vi "Untitled 1.vi"() -> ()   [LabVIEW 2024]
uses:
  <vilib>/DAQmx/read.llb/DAQmx Read (Analog 1D Wfm NChan NSamp).vi
  <vilib>/addons/database/Connection.llb/DB Tools Open Connec (Path).vi
  <vilib>/Utility/file.llb/Write Delimited Spreadsheet (DBL).vi
  <vilib>/DAQmx/miscellaneous.llb/DAQmx Fill In Error Info.vi
  <vilib>/addons/database/NI_Database_API.lvlib
panel:
  out "overflow element":dbl[][](array[numeric])
  out "error out":errorcluster
  in  "connection information":path
  in  "stop":bool
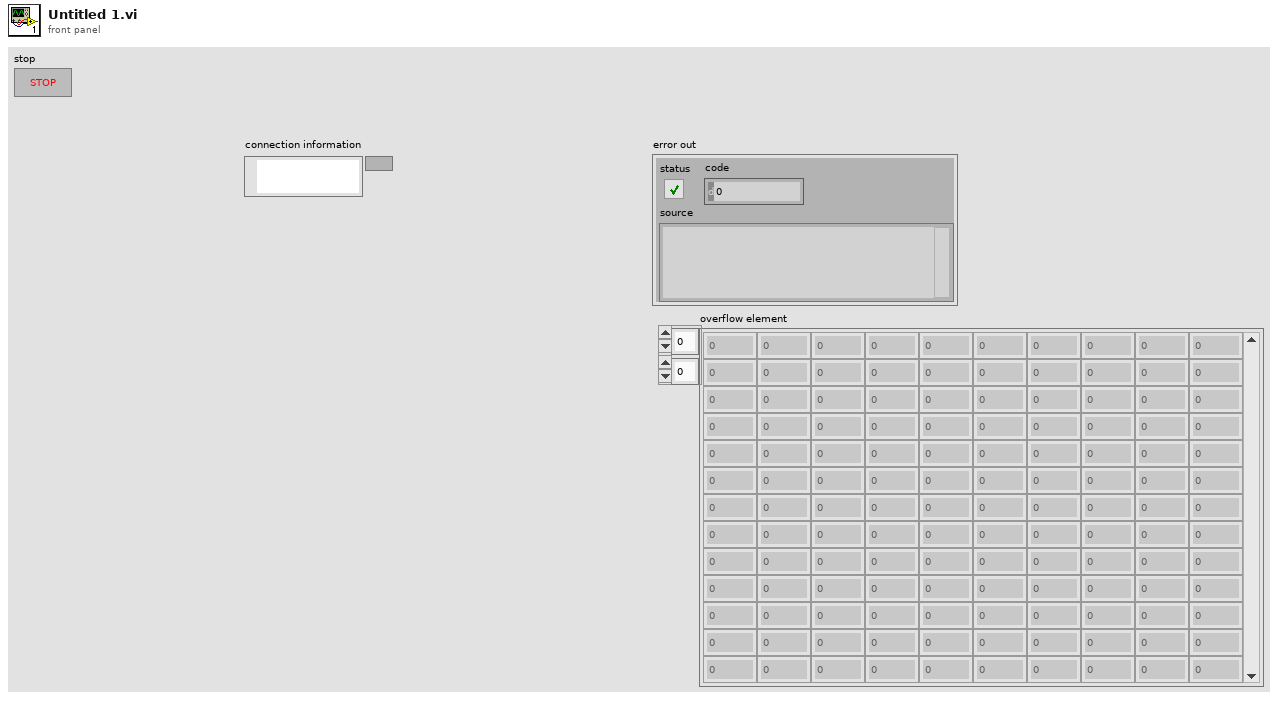
[diagram p1: front panel]
types:
  T1 = typedef "NI_Database_API.lvlib/Conn ObjectReference.ctl" = refnum<k1>
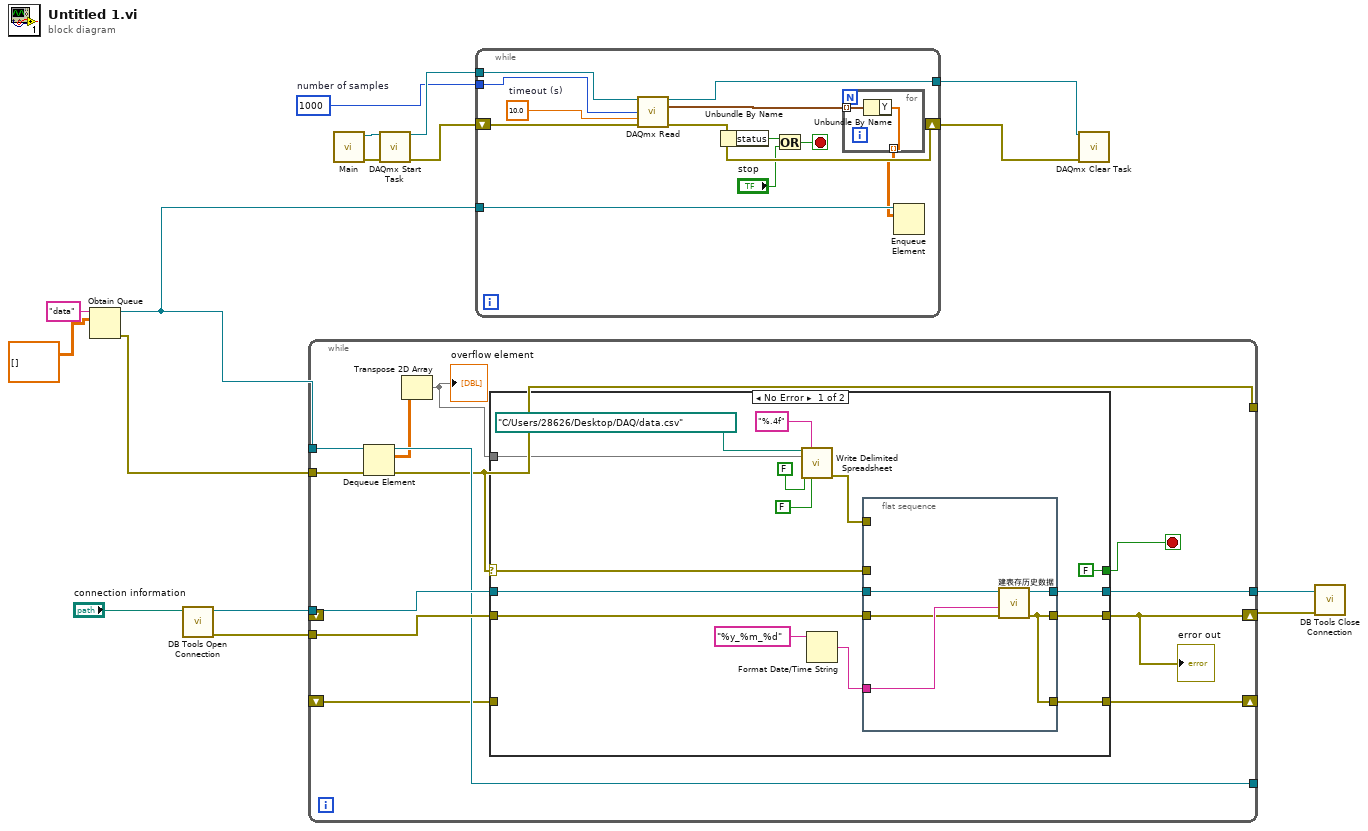
[diagram p0: block diagram]
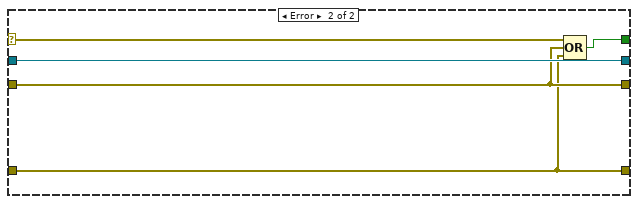
[diagram p2: hidden frame]
diagram:
  w14 = 1000  # number of samples
  n1 = Obtain Queue(name (unnamed)="data", element data type=dbl[][] [] ("appended array")) -> (queue out=w4:refnum<queue>, error out=w1:errorcluster)  [unwired: 3 in, 1 out]
  n2 = call-poly <vilib>:"DB Tools Open Connection.vi"("connection information"="connection information") -> ("error out"=w8:errorcluster, "connection reference"=w7:T1)  [unwired: 7 in]
  n3 = while {
    tunnel: w8 -> [w29]
    tunnel: w7 -> [w28]
    tunnel: w4 -> [w27]
    tunnel: [w26] -> _
    tunnel: [w24] -> w5
    shift-right: [w21] -> w6
    shift-left: _ -> [_]
    shift-right: [w25] -> _
    shift-left: _ -> [w23]
    tunnel: w1 -> [w20]
    tunnel: [w19] -> _
    stop <- w22 stop-if-true
    n4 = Dequeue Element(queue=w27, error in (no error)=w20) -> (queue out=w26:refnum<queue>, element=w18:dbl[][], error out=w19:errorcluster)  [unwired: 1 in, 1 out]
    n5 = Transpose 2D Array(2D array=w18) -> (transposed array=w17:dbl[][])
    "overflow element" <- w17
    n6 = case shown="No Error" w19 {
      selector: w19 -> [w44 w53]
      tunnel: [FALSE w51] -> w22
      tunnel: w28 -> [w43 w54]
      tunnel: w29 -> [w42 w52]
      tunnel: [w41 w54] -> w24
      tunnel: [w40 w52] -> w21
      tunnel: [w33 w50] -> w25
      tunnel: w23 -> [_ w50]
      tunnel: w17 -> [w31 _]
      frame No Error {
        n7 = call-poly <vilib>:"Write Delimited Spreadsheet.vi"("file path (dialog if empty)"=path "C:/Users/28626/Desktop/DAQ/data.csv", "format (%.3f)"="%.4f", "2D data"=w31, "append to file? (new file:F)"=FALSE, "transpose? (no:F)"=FALSE) -> ("error out"=w39:errorcluster)  [unwired: 9 in, 1 out]
        n8 = Format Date/Time String(time format string (%c)="%y_%m_%d") -> (date/time string=w34:string)  [unwired: 2 in]
        n9 = flat-sequence {
          tunnel: w44 -> [_]
          tunnel: w43 -> [w48]
          tunnel: w42 -> [w47]
          tunnel: [w46] -> w41
          tunnel: [w45] -> w40
          tunnel: w39 -> [_]
          tunnel: w34 -> [w49]
          tunnel: [w45] -> w33
          frame #0 {
            n10 = call "建表存历史数据.vi"("error in (no error)"=w47, "表名"=w49, "connection reference"=w48) -> ("error out"=w45:errorcluster, "connection reference 2"=w46:T1)  [unwired: 7 in]
          }
        }
      }
      frame Error {
        n11 = Compound Arithmetic op=OR(w53, w52, w50) -> (w51:bool)
      }
    }
    "error out" <- w21
  }
  n12 = call "Main.vi"() -> ("error out"=w10:errorcluster, "task out"=w11:refnum<k21>)  [unwired: 10 in]
  n13 = call <vilib>:"DAQmx Start Task.vi"("task/channels in"=w11, "error in"=w10) -> ("task out"=w16:refnum<k21>, "error out"=w15:errorcluster)  [unwired: 12 in]
  n14 = while {
    tunnel: w16 -> [w66]
    tunnel: w14 -> [w63]
    tunnel: [w64] -> w12
    shift-right: [w61] -> w13
    shift-left: w15 -> [w65]
    tunnel: w4 -> [w57]
    stop <- w60 stop-if-true
    w58 = 10.0  # timeout (s)
    n15 = call-poly <vilib>:"DAQmx Read.vi"("task/channels in"=w66, "number of samples per channel"=w63, "timeout"=w58, "error in"=w65) -> ("task out"=w64:refnum<k21>, "data"=w56:waveform(dbl)[], "error out"=w61:errorcluster)  [unwired: 9 in]
    n16 = Unbundle By Name(w61) -> ("status"=w62:bool)
    n17 = Or(x=w62, y="stop") -> (x .or. y?=w60:bool)
    n18 = for {
      tunnel: w56 -> [w68] mode=indexing
      tunnel: [w67] -> w55 mode=indexing
      n19 = Unbundle By Name(w68) -> ("Y"=w67:dbl[])
    }
    n20 = Enqueue Element(queue=w57, element=w55) -> ()  [unwired: 2 in, 3 out]
  }
  n21 = call <vilib>:"DAQmx Clear Task.vi"("task in"=w12, "error in"=w13) -> ()  [unwired: 13 in, 1 out]
  n22 = call <vilib>:"DB Tools Close Connection.vi"("error in (no error)"=w6, "connection reference"=w5) -> ()  [unwired: 5 in, 1 out]
